vi "GetAllObjectData.vi"(8 "ErrorIn":errorcluster, 11 "ReferenceIn":refnum<class "IApplicationConfiguration.lvclass">) -> (0 "ErrorOut":errorcluster, 2 "Objects":T1[](array[typedef]), 3 "ReferenceOut":refnum<class "IApplicationConfiguration.lvclass">)   [LabVIEW 2021, in "IApplicationConfiguration.lvclass"]
uses:
  IApplicationConfiguration.lvclass
  ObjectDataDetails.ctl
  ObjectData.ctl
panel:
  # "e"
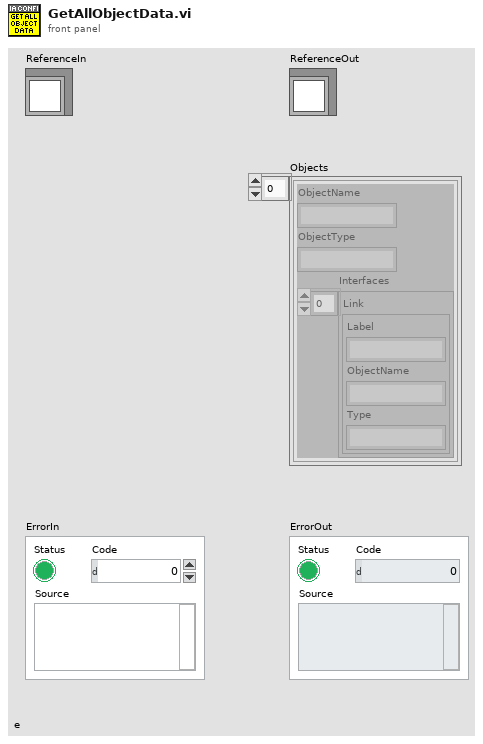
[diagram p1: front panel]
types:
  T1 = typedef "IApplicationConfiguration.lvclass/ObjectDataDetails.ctl" = cluster{"ObjectName":string, "ObjectType":string, "Interfaces":T2[]}
  T2 = typedef "IApplicationConfiguration.lvclass/ObjectData.ctl" = cluster{"Label":string, "ObjectName":string, "Type":string}
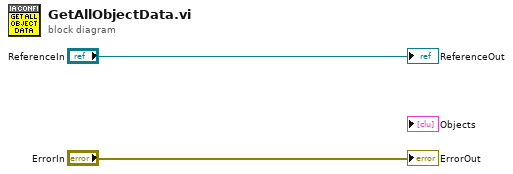
[diagram p0: block diagram]
diagram:
  "ErrorOut" <- "ErrorIn"
  "ReferenceOut" <- "ReferenceIn"
